vi "niTuner Set Freq.vi"   [LabVIEW 2011]
doc: "This polymorphic VI is capable of tuning the PXI-5600 to up to 720 center frequencies in sequence using a scan list. If you are using only a single scan list entry, you can use the Set Freq(f) version of this VI, but if there is more than one entry in the scan list you must use the Set Freq (f array) version. To select the Set Freq (f array) version, right-click on the Set Freq icon in your block diagram and click <B>select type»Set Freq (f array).vi.</B>"
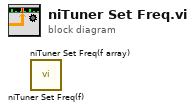
[diagram p0: block diagram]
diagram:
  n1 = call <instrlib>:"niTuner Set Freq(f).vi"() -> ()  [unwired: 7 in, 5 out]
  n2 = call <instrlib>:"niTuner Set Freq(f array).vi"() -> ()  [unwired: 7 in, 5 out]
